vi "Instrument fgv.vi"(7 "Enum":T1(ring), 8 "error in (no error) 2":errorcluster, 10 "WriteCC1":string[](array[string])=[""], 11 "INPUT":T2) -> (0 "error":errorcluster, 2 "WriteCC1 2":string[](array[string]), 3 "output":T2)   [LabVIEW 2025]
uses:
  <vilib>/Instr/_visa.llb/VISA Configure Serial Port (Instr).vi
panel:
  out "error out 3":errorcluster
  out "error out 2":errorcluster
  out "error out":errorcluster
  out "Serial Settings:Number of Bytes at Serial Port":u32
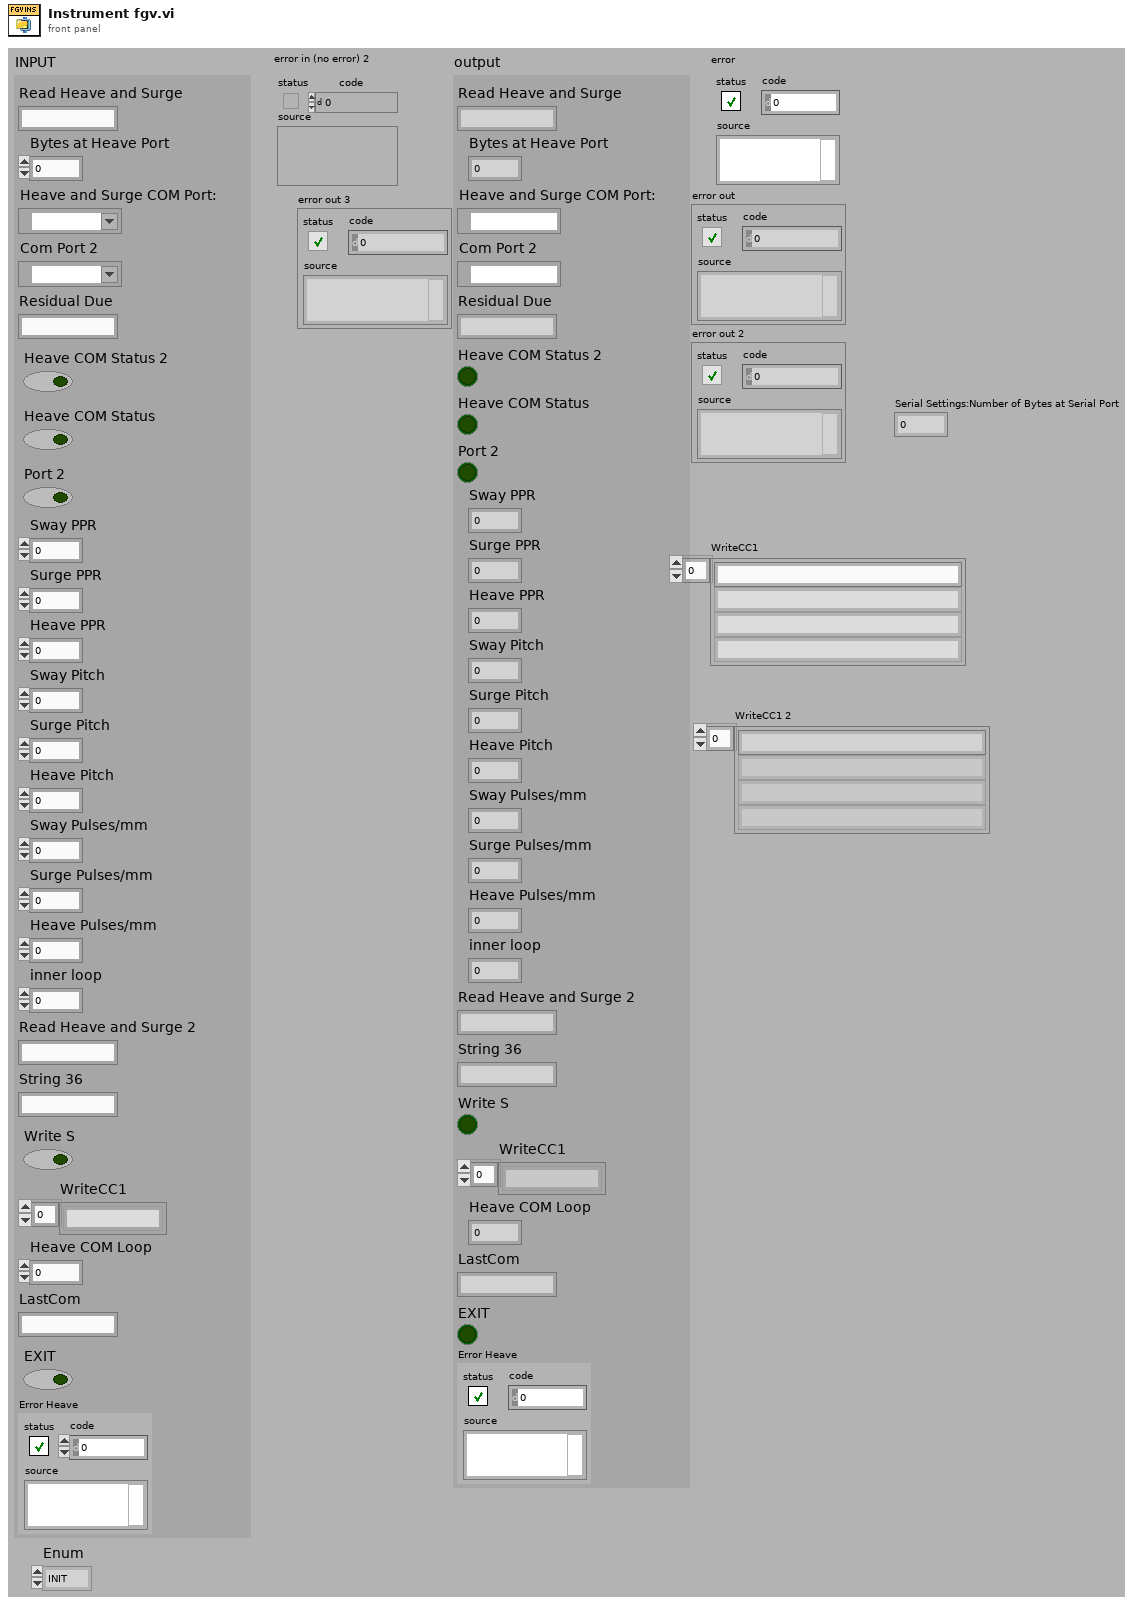
[diagram p1: front panel]
types:
  T1 = enum16{"INIT", "READ", "MANUAL WRITE", "WRITE", "CLOSE", "ERROR INIT"}
  T2 = cluster{"Read Heave and Surge":string, "Bytes at Heave Port":dbl, "Heave and Surge COM Port:":refnum<visa-resource-name>, "Com Port 2":refnum<visa-resource-name>, "Residual Due":string, "Heave COM Status 2":bool, "Heave COM Status":bool, "Port 2":bool, "Sway PPR":dbl, "Surge PPR":dbl, "Heave PPR":dbl, "Sway Pitch":dbl, "Surge Pitch":dbl, "Heave Pitch":dbl, "Sway Pulses/mm":dbl, "Surge Pulses/mm":dbl, "Heave Pulses/mm":dbl, "inner loop":dbl, "Read Heave and Surge 2":string, "String 36":string, "Write S":bool, "WriteCC1":string[], "Heave COM Loop":i32, "LastCom":string, "EXIT":bool, "Error Heave":errorcluster}
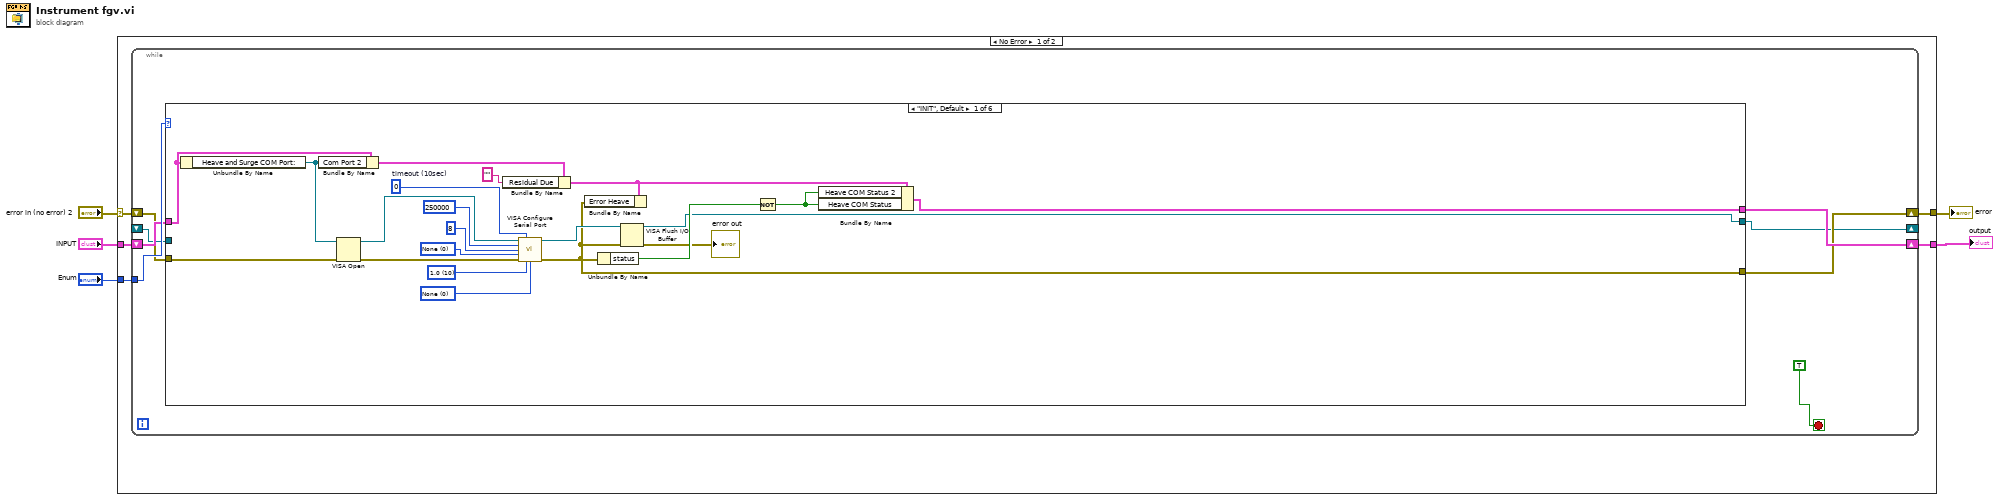
[diagram p0: block diagram]
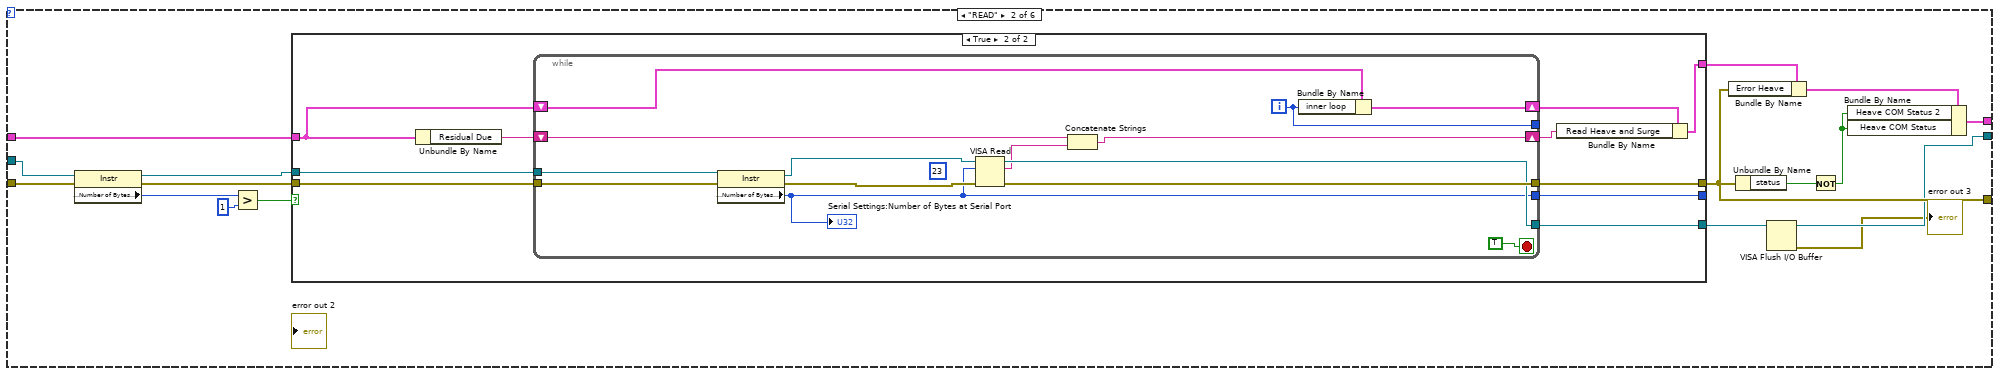
[diagram p2: hidden frame]
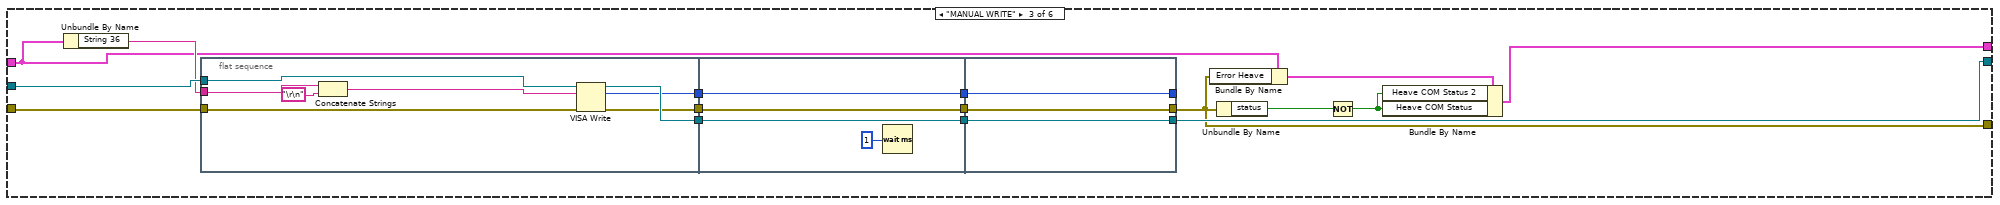
[diagram p4: hidden frame]
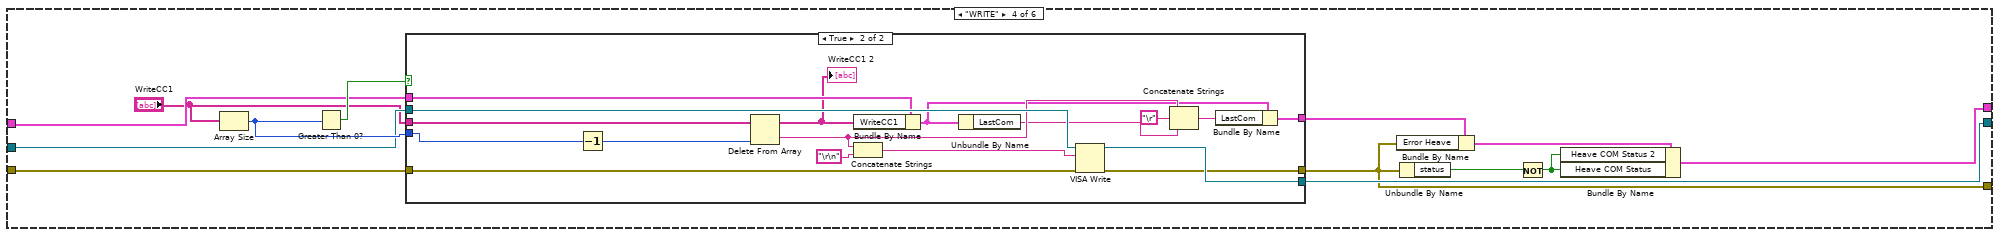
[diagram p5: hidden frame]
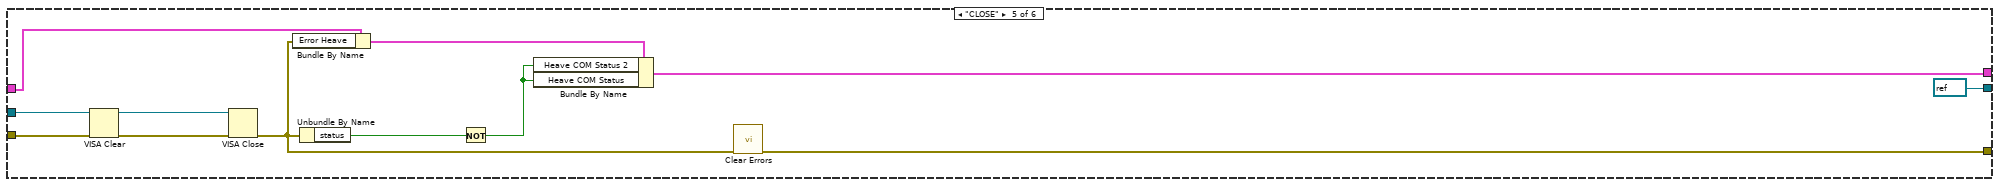
[diagram p7: hidden frame]
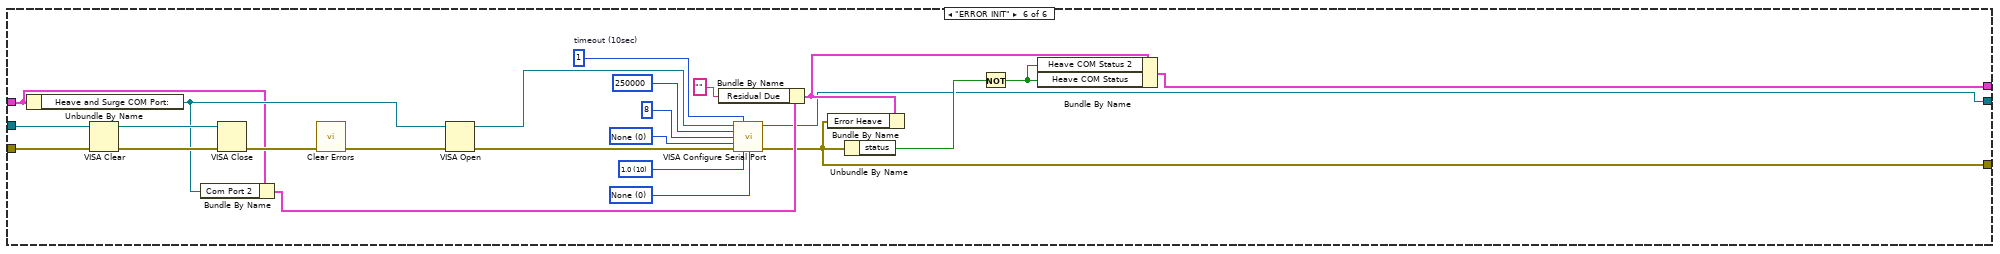
[diagram p8: hidden frame]
diagram:
  n1 = case shown="No Error" "error in (no error) 2" {
    selector: "error in (no error) 2" -> [w9 w184]
    tunnel: [w10 w184] -> w2
    tunnel: "Enum" -> [w8 _]
    tunnel: "INPUT" -> [w7 w185]
    tunnel: [w6 w185] -> w5
    frame No Error {
      n2 = while {
        tunnel: w8 -> [w17]
        shift-right: [w13] -> w10
        shift-left: w9 -> [w14]
        shift-right: [w16] -> w6
        shift-left: w7 -> [w15]
        shift-right: [w12] -> _
        shift-left: _ -> [w11]
        stop <- TRUE ("stop 3") stop-if-true
        n3 = case shown="\"INIT\", Default" w17 {
          tunnel: [w28 w45 w85 w119 w149 w160] -> w16
          tunnel: w15 -> [w24 w49 w87 w122 w150 w164]
          tunnel: w14 -> [w25 w56 w91 w124 w157 w180]
          tunnel: [w20 w43 w86 w118 w155 w162] -> w13
          tunnel: [w21 w41 w92 w123 refnum<visa-resource-name> refnum ("duplicate VISA resource name") w161] -> w12
          tunnel: w11 -> [_ w55 w93 w125 w156 w179]
          frame "INIT", Default {
            w38 = u16 0 items=["None", "XON/XOFF", "RTS/CTS", "XON/XOFF & RTS/CTS", "DTR/DSR", "XON/XOFF & DTR/DSR"] ("flow control (0:none)  2")
            w36 = u16 10 items=["1.0"=10, "1.5"=15, "2.0"=20] ("stop bits 2")
            w35 = u16 0 items=["None", "Odd", "Even", "Mark", "Space"] ("parity 2")
            w33 = u32 0  # timeout (10sec)
            n4 = Unbundle By Name(w24) -> ("Heave and Surge COM Port:"=w22:refnum<visa-resource-name>)
            n5 = Bundle By Name(cluster=w24, "Com Port 2"=w22) -> (w23:T2)
            n6 = VISA Open(error in (no error)=w25, VISA resource name=w22) -> (VISA resource name=w31:refnum<visa-resource-name>, error out=w32:errorcluster)  [unwired: 3 in]
            n7 = Bundle By Name(cluster=w23, "Residual Due"="") -> (w29:T2)
            n8 = call-poly "VISA Configure Serial Port"("VISA resource name"=w31, "timeout (10sec)"=w33, "baud rate (9600)"=u32 250000 ("baud rate  2"), "data bits (8)"=u16 8 ("data bits  2"), "parity (0:none)"=w35, "error in (no error)"=w32, "stop bits (10: 1 bit)"=w36, "flow control (0:none)"=w38) -> ("VISA resource name out"=w30:refnum<visa-resource-name>, "error out"=w20:errorcluster)  [unwired: 6 in]
            n9 = Bundle By Name(cluster=w29, "Error Heave"=w20) -> ()  [unwired: 1 out]
            n10 = Unbundle By Name(w20) -> ("status"=w27:bool)
            n11 = VISA Flush I/O Buffer(VISA resource name=w30, error in (no error)=w20) -> (VISA resource name out=w21:refnum<visa-resource-name>, error out=→"error out":errorcluster)  [unwired: 1 in]
            n12 = Not(x=w27) -> (.not. x?=w26:bool)
            n13 = Bundle By Name(cluster=w29, "Heave COM Status 2"=w26, "Heave COM Status"=w26) -> (w28:T2)
          }
          frame "READ" {
            n14 = property class="Instr"(reference=w55, error in=w56) -> (reference out=w51:refnum<visa-resource-name>, error out=w50:errorcluster, "Serial Settings:Number of Bytes at Serial Port"=w54:u32)
            n15 = Greater?(x=w54, y=u32 1) -> (0:w52:bool)
            n16 = case shown="True" w52 {
              tunnel: w51 -> [w59 w66]
              tunnel: w50 -> [w58 w67]
              tunnel: [w58 w69] -> w43
              tunnel: [w59 w68] -> w42
              tunnel: w49 -> [w57 w65]
              tunnel: [w57 w62] -> w48
              tunnel: [_ w60] -> _
              frame False {
              }
              frame True {
                n17 = Unbundle By Name(w65) -> ("Residual Due"=w64:string)
                n18 = while {
                  tunnel: [w81] -> w69
                  tunnel: [w80] -> w68
                  tunnel: w67 -> [w79]
                  tunnel: w66 -> [w78]
                  tunnel: [w72] -> _
                  shift-right: [w77] -> w61
                  shift-left: w64 -> [w76]
                  shift-right: [w73] -> w63
                  shift-left: w65 -> [w74]
                  tunnel: [w70] -> w60
                  i -> [w72]
                  stop <- TRUE stop-if-true
                  (unwired) u32 23 ("byte count")
                  n19 = property class="Instr"(reference=w78, error in=w79) -> (reference out=w83:refnum<visa-resource-name>, error out=w82:errorcluster, "Serial Settings:Number of Bytes at Serial Port"=w70:u32)
                  "Serial Settings:Number of Bytes at Serial Port" <- w70
                  n20 = VISA Read(VISA resource name=w83, byte count=w70, error in (no error)=w82) -> (VISA resource name out=w80:refnum<visa-resource-name>, read buffer=w75:string, error out=w81:errorcluster)  [unwired: 1 out]
                  n21 = Concatenate Strings(w76, w75) -> (w77:string)
                  n22 = Bundle By Name(cluster=w74, "inner loop"=w72) -> (w73:T2)
                }
                n23 = Bundle By Name(cluster=w63, "Read Heave and Surge"=w61) -> (w62:T2)
              }
            }
            n24 = Bundle By Name(cluster=w48, "Error Heave"=w43) -> (w47:T2)
            n25 = Unbundle By Name(w43) -> ("status"=w46:bool)
            n26 = VISA Flush I/O Buffer(VISA resource name=w42) -> (VISA resource name out=w41:refnum<visa-resource-name>, error out=→"error out 3":errorcluster)  [unwired: 2 in]
            n27 = Not(x=w46) -> (.not. x?=w44:bool)
            n28 = Bundle By Name(cluster=w47, "Heave COM Status 2"=w44, "Heave COM Status"=w44) -> (w45:T2)
          }
          frame "MANUAL WRITE" {
            n29 = Unbundle By Name(w87) -> ("String 36"=w90:string)
            n30 = flat-sequence {
              tunnel: w93 -> [w104]
              tunnel: w91 -> [w103]
              tunnel: w90 -> [w102]
              tunnel: [w107] -> w99
              tunnel: [w106] -> w98
              tunnel: [w105] -> w97
              tunnel: w99 -> [w111]
              tunnel: w98 -> [w110]
              tunnel: w97 -> [w109]
              tunnel: [w111] -> w96
              tunnel: [w110] -> w95
              tunnel: [w109] -> w94
              tunnel: [w112] -> _
              tunnel: [w113] -> w86
              tunnel: [w114] -> w92
              tunnel: w96 -> [w114]
              tunnel: w95 -> [w113]
              tunnel: w94 -> [w112]
              frame #0 {
                n31 = Concatenate Strings(w102, "\r\n") -> (w101:string)
                n32 = VISA Write(VISA resource name=w104, write buffer=w101, error in (no error)=w103) -> (VISA resource name out=w107:refnum<visa-resource-name>, return count=w105:u32, error out=w106:errorcluster)
              }
              frame #1 {
                n33 = Wait (ms)(milliseconds to wait=u32 1) -> ()  [unwired: 1 out]
              }
              frame #2 {
              }
            }
            n34 = Bundle By Name(cluster=w87, "Error Heave"=w86) -> (w89:T2)
            n35 = Unbundle By Name(w86) -> ("status"=w88:bool)
            n36 = Not(x=w88) -> (.not. x?=w84:bool)
            n37 = Bundle By Name(cluster=w89, "Heave COM Status 2"=w84, "Heave COM Status"=w84) -> (w85:T2)
          }
          frame "WRITE" {
            n38 = Array Size(array="WriteCC1") -> (size(s)=w127:i32)
            n39 = Greater Than 0?(x=w127) -> (x > 0?=w126:bool)
            n40 = case shown="True" w126 {
              tunnel: [w130 w140] -> w118
              tunnel: w124 -> [w130 w146]
              tunnel: [w129 w144] -> w123
              tunnel: w125 -> [w129 w145]
              tunnel: "WriteCC1" -> [_ w141]
              tunnel: w127 -> [_ w143]
              tunnel: w122 -> [w128 w137]
              tunnel: [w128 w134] -> w121
              frame False {
              }
              frame True {
                n41 = Decrement(x=w143) -> (x-1=w142:i32)
                n42 = Delete From Array(array=w141, index=w142) -> (deleted portion=w139:string, array with subset deleted=w133:string[])  [unwired: 1 in]
                "WriteCC1 2" <- w133
                n43 = Bundle By Name(cluster=w137, "WriteCC1"=w133) -> (w136:T2)
                n44 = Concatenate Strings(w139, "\r\n") -> (w132:string)
                n45 = Unbundle By Name(w136) -> ("LastCom"=w135:string)
                n46 = VISA Write(VISA resource name=w145, write buffer=w132, error in (no error)=w146) -> (VISA resource name out=w144:refnum<visa-resource-name>, error out=w140:errorcluster)  [unwired: 1 out]
                n47 = Concatenate Strings(w139, "\r", w135) -> (w138:string)
                n48 = Bundle By Name(cluster=w136, "LastCom"=w138) -> (w134:T2)
              }
            }
            n49 = Bundle By Name(cluster=w121, "Error Heave"=w118) -> (w120:T2)
            n50 = Unbundle By Name(w118) -> ("status"=w117:bool)
            n51 = Not(x=w117) -> (.not. x?=w116:bool)
            n52 = Bundle By Name(cluster=w120, "Heave COM Status 2"=w116, "Heave COM Status"=w116) -> (w119:T2)
          }
          frame "CLOSE" {
            n53 = VISA Clear(VISA resource name=w156, error in (no error)=w157) -> (VISA resource name out=w159:refnum<visa-resource-name>, error out=w158:errorcluster)
            n54 = VISA Close(VISA resource name=w159, error in (no error)=w158) -> (error out=w151:errorcluster)
            n55 = Bundle By Name(cluster=w150, "Error Heave"=w151) -> (w154:T2)
            n56 = Unbundle By Name(w151) -> ("status"=w153:bool)
            n57 = Not(x=w153) -> (.not. x?=w152:bool)
            n58 = Bundle By Name(cluster=w154, "Heave COM Status 2"=w152, "Heave COM Status"=w152) -> (w149:T2)
            n59 = call <vilib>:"Clear Errors.vi"("error in (no error)"=w151) -> ("error out"=w155:errorcluster)  [unwired: 5 in, 1 out]
          }
          frame "ERROR INIT" {
            w177 = u16 0 items=["None", "XON/XOFF", "RTS/CTS", "XON/XOFF & RTS/CTS", "DTR/DSR", "XON/XOFF & DTR/DSR"] ("flow control (0:none)  2")
            w175 = u16 10 items=["1.0"=10, "1.5"=15, "2.0"=20] ("stop bits 2")
            w174 = u16 0 items=["None", "Odd", "Even", "Mark", "Space"] ("parity 2")
            w172 = u32 1  # timeout (10sec)
            n60 = Unbundle By Name(w164) -> ("Heave and Surge COM Port:"=w165:refnum<visa-resource-name>)
            n61 = VISA Clear(VISA resource name=w179, error in (no error)=w180) -> (VISA resource name out=w183:refnum<visa-resource-name>, error out=w182:errorcluster)
            n62 = Bundle By Name(cluster=w164, "Com Port 2"=w165) -> (w166:T2)
            n63 = VISA Close(VISA resource name=w183, error in (no error)=w182) -> (error out=w181:errorcluster)
            n64 = call <vilib>:"Clear Errors.vi"("error in (no error)"=w181) -> ("error out"=w163:errorcluster)  [unwired: 5 in, 1 out]
            n65 = VISA Open(error in (no error)=w163, VISA resource name=w165) -> (VISA resource name=w170:refnum<visa-resource-name>, error out=w171:errorcluster)  [unwired: 3 in]
            n66 = Bundle By Name(cluster=w166, "Residual Due"="") -> (w169:T2)
            n67 = call-poly "VISA Configure Serial Port"("VISA resource name"=w170, "timeout (10sec)"=w172, "baud rate (9600)"=u32 250000 ("baud rate  2"), "data bits (8)"=u16 8 ("data bits  2"), "parity (0:none)"=w174, "error in (no error)"=w171, "stop bits (10: 1 bit)"=w175, "flow control (0:none)"=w177) -> ("VISA resource name out"=w161:refnum<visa-resource-name>, "error out"=w162:errorcluster)  [unwired: 6 in]
            n68 = Bundle By Name(cluster=w169, "Error Heave"=w162) -> ()  [unwired: 1 out]
            n69 = Unbundle By Name(w162) -> ("status"=w168:bool)
            n70 = Not(x=w168) -> (.not. x?=w167:bool)
            n71 = Bundle By Name(cluster=w169, "Heave COM Status 2"=w167, "Heave COM Status"=w167) -> (w160:T2)
          }
        }
      }
    }
    frame Error {
    }
  }
  "output" <- w5
  "error" <- w2
